vi "Find Duplicate Series.vi"() -> ()   [LabVIEW 2024]
panel:
  out "Array":cluster{"value":path, "Folder Path":path}[](array[cluster])
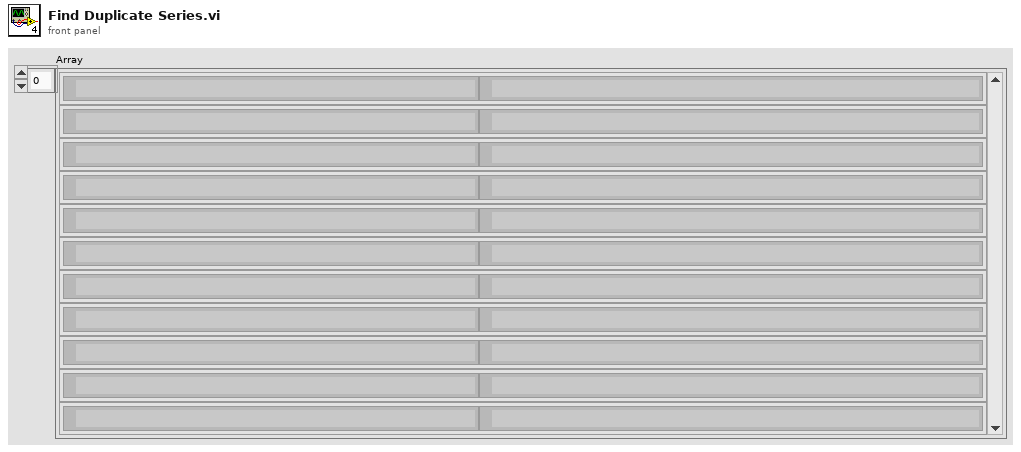
[diagram p1: front panel]
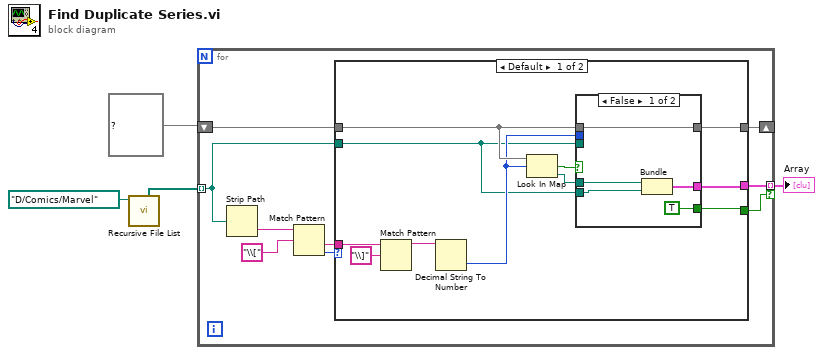
[diagram p0: block diagram]
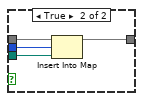
[diagram p2: hidden frame]
diagram:
  n1 = call <vilib>:"Recursive File List.vi"("Folder Path"=path "D:/Comics/Marvel") -> ("All Folders"=w3:path[])  [unwired: 6 in, 4 out]
  n2 = for {
    tunnel: w3 -> [w7] mode=indexing
    shift-right: [w8] -> _
    shift-left: map{i32, path} {} ("map") -> [w9]
    tunnel: [w6] -> w1 mode=indexing if=w5
    n3 = Strip Path(path=w7) -> (name=w13:string)  [unwired: 1 out]
    n4 = Match Pattern(string=w13, regular expression="\\[") -> (after substring=w10:string, offset past match=w11:i32)  [unwired: 1 in, 2 out]
    n5 = case shown="Default" w11 {
      tunnel: w10 -> [w24 _]
      tunnel: w9 -> [w21 w34]
      tunnel: [w18 w34] -> w8
      tunnel: w7 -> [w16 _]
      tunnel: [w15 _] -> w6
      tunnel: [w14 _] -> w5
      frame Default {
        n6 = Match Pattern(string=w24, regular expression="\\]") -> (before substring=w22:string)  [unwired: 1 in, 3 out]
        n7 = Decimal String To Number(string=w22) -> (number=w20:i32)  [unwired: 2 in, 1 out]
        n8 = Look In Map(map=w21, key=w20) -> (key not found?=w19:bool, value=w17:path)  [unwired: 1 in]
        n9 = case shown="False" w19 {
          tunnel: w16 -> [_ w33]
          tunnel: w21 -> [w29 w32]
          tunnel: w20 -> [_ w31]
          tunnel: [w29 w30] -> w18
          tunnel: w17 -> [w28 _]
          tunnel: w16 -> [w27 _]
          tunnel: [w26 _] -> w15
          tunnel: [TRUE _] -> w14
          frame False {
            n10 = Bundle("value"=w28, "Folder Path"=w27) -> (w26:cluster{"value":path, "Folder Path":path})  [unwired: 1 in]
          }
          frame True {
            n11 = Insert Into Map(map in=w32, key=w31, value=w33) -> (map out=w30:map{i32, path})  [unwired: 2 out]
          }
        }
      }
      frame -1 {
      }
    }
  }
  "Array" <- w1
